vi "Send Write Main MSG.vi"(11 "Controller in":refnum<class "Controller.lvclass">) -> ()   [LabVIEW 2014, in "Controller.lvlib" / "Controller.lvclass"]
uses:
  Controller.lvclass
  Controller.lvclass/Controller.ctl
  <vilib>/Platform/TimedLoop/XDataNode/timing_clust.ctl
  <vilib>/Platform/TimedLoop/XDataNode/nitl_modes.ctl
  <vilib>/Platform/TimedLoop/XDataNode/wakeup.ctl
  File Actor/Messages/To/Data/File Data Message.lvclass
  Controls/eMap.ctl
  <vilib>/ActorFramework/Message Enqueuer/Message Enqueuer.lvclass
  reusable/Data/Data.lvclass
  File Actor/Messages/To/Data/File Data Message.lvclass/File Data Message.ctl
  <vilib>/ActorFramework/Message Enqueuer/Message Enqueuer.lvclass/Message Enqueuer.ctl
  <vilib>/ActorFramework/Message Priority Queue/Priority Enqueue.vi
  <vilib>/Platform/TimedLoop/XDataNode/XDataNode.xnode
  <vilib>/Platform/TimedLoop/XDataNode/XDNodeRunTimeDep.lvlib
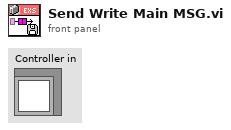
[diagram p1: front panel]
types:
  T1 = typedef "XDNodeRunTimeDep.lvlib/timing_clust.ctl" = cluster{"Expected End [f-1]":u64, "Actual End [f-1]":u64, "Finished Late? [f-1]":bool, "Expected End [i-1]":u64, "Actual End [i-1]":u64, "Finished Late? [i-1]":bool, "Expected Start [i]":u64, "Actual Start [i]":u64, "Expected Start [f]":u64, "Actual Start [f]":u64, "Source Name":string, "Structure Name":string, "Period":i64, "Deadline":i64, "Offset":i64, "Start":i64, "Priority":i32, "Timeout":i32, "Mode":T2, "Wakeup Reason":T3, "Error":errorcluster, "Source Type":string, "Secondary Source Type":string, "Global End Time":u64, "Global Start Time":u64, "Frame Duration":u64, "Iteration Duration":u64, "Assigned CPU":i32, "I/O Scan Engine Mode":u32}
  T2 = typedef "XDNodeRunTimeDep.lvlib/nitl_modes.ctl" = enum32{"No Change", "Process missed periods, maintain original phase", "Discard missed periods, maintain original phase", "Process missed periods, ignore original phase", "Discard missed periods, ignore original phase"}
  T3 = typedef "XDNodeRunTimeDep.lvlib/wakeup.ctl" = enum32{"Normal", "Aborted", "Asynchronous wakeup", "Timing source error", "Timed loop error", "Timeout"}
  T4 = typedef "Controller.lvlib/Controller.lvclass/eMap.ctl" = cluster{"Enqueuer":refnum<class "Message Enqueuer.lvclass">, "Active":bool}
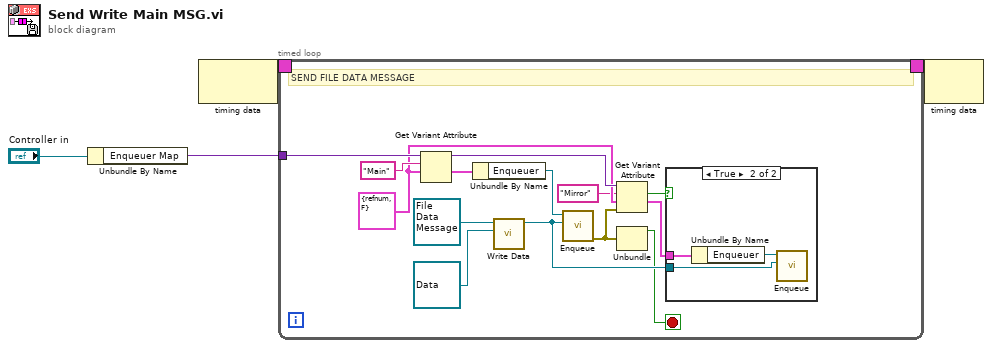
[diagram p0: block diagram]
diagram:
  n1 = Unbundle By Name("Controller in") -> ("Enqueuer Map"=w1:variant)
  n2 = node-c288() -> (w4:T1)  [unwired: 1 in]
  n3 = timed-loop {
    timing: w4 -> [_]
    timing-out: [_] -> w3
    tunnel: w1 -> [w17]
    stop <- w10 stop-if-true
    w12 = T4 {"Enqueuer"=refnum, "Active"=FALSE} ("eMap")
    # "SEND FILE DATA MESSAGE"
    n4 = Get Variant Attribute(Variant=w17, name="Main", default value (empty Variant)=w12) -> (duplicate Variant=w13:variant, value=w16:T4)  [unwired: 1 in, 2 out]
    n5 = Unbundle By Name(w16) -> ("Enqueuer"=w15:refnum<class "Message Enqueuer.lvclass">)
    n6 = call "Write Data.vi"("Base Data Lib:Data"=refnum<class "Data.lvclass"> refnum, "File Data Message in"=refnum<class "File Data Message.lvclass"> refnum ("File Library.lvlib:File Data MSG")) -> ("File Data Message out"=w11:refnum<class "File Data Message.lvclass">)  [unwired: 8 in, 1 out]
    n7 = call <vilib>:"Enqueue.vi"("Message"=w11, "Message Enqueuer in"=w15) -> ("error out"=w5:errorcluster)  [unwired: 8 in, 1 out]
    n8 = Get Variant Attribute(Variant=w13, name="Mirror", default value (empty Variant)=w12, error in=w5) -> (found=w7:bool, value=w6:T4)  [unwired: 2 out]
    n9 = Unbundle(w5) -> ("status"=w10:bool)  [unwired: 2 out]
    n10 = case shown="True" w7 {
      tunnel: w6 -> [_ w21]
      tunnel: w11 -> [_ w19]
      frame False {
      }
      frame True {
        n11 = Unbundle By Name(w21) -> ("Enqueuer"=w20:refnum<class "Message Enqueuer.lvclass">)
        n12 = call <vilib>:"Enqueue.vi"("Message"=w19, "Message Enqueuer in"=w20) -> ()  [unwired: 8 in, 2 out]
      }
    }
  }
  n13 = node-c288(w3) -> ()  [unwired: 1 out]
